vi "Host_XYConstantCurrent.vi"() -> ()   [LabVIEW 2014]
uses:
  <vilib>/FPGAPlugInAG/PCIe-7851R/niLvFpga_Open_PCIe-7851R.vi
  <vilib>/rvi/interface/common/dynamic/niFpgaDynamicAddResources.vi
  <vilib>/Utility/error.llb/Error Cluster From Error Code.vi
  <vilib>/rvi/errors/niLvFpgaAdjustHostInterfaceError.vi
  <vilib>/FPGAPlugInAG/Dynamic/niLvFpga_Close_Dynamic.vi
  <vilib>/rvi/interface/nirviOpenFPGA/nirviOpenFPGA.xnode
  FPGA Bitfiles/PCCrossingXYProj_FPGATarget_FPGAXYMoving_0UyQVClWLPs.lvbitx
  <vilib>/rvi/interface/nirviReadWriteControl/nirviReadWriteControl.xnode
  <vilib>/rvi/interface/nirviCloseFPGA/nirviCloseFPGA.xnode
  NiFpgaLv.dll
  <vilib>/rvi/interface/Simulation/niFpgaSimulationCallBeginRW.vi
panel:
  out "YPresNum":i32
  out "XPresNum":i32
  in  "stop":bool
  in  "YOffset":i16
  in  "XOffset":i16
  in  "YStepLen":i16
  in  "XStepLen":i16
  in  "YNum":i16
  in  "XNum":i16
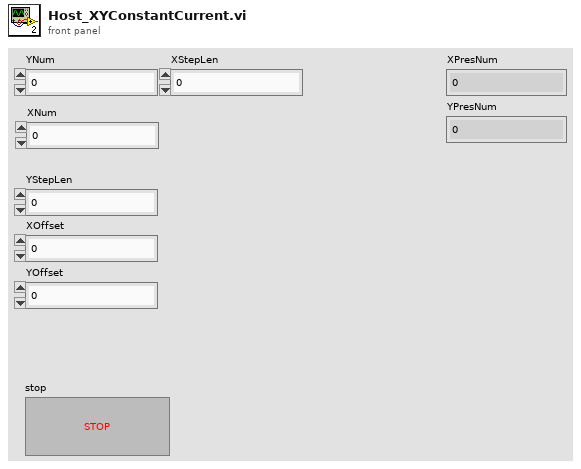
[diagram p1: front panel]
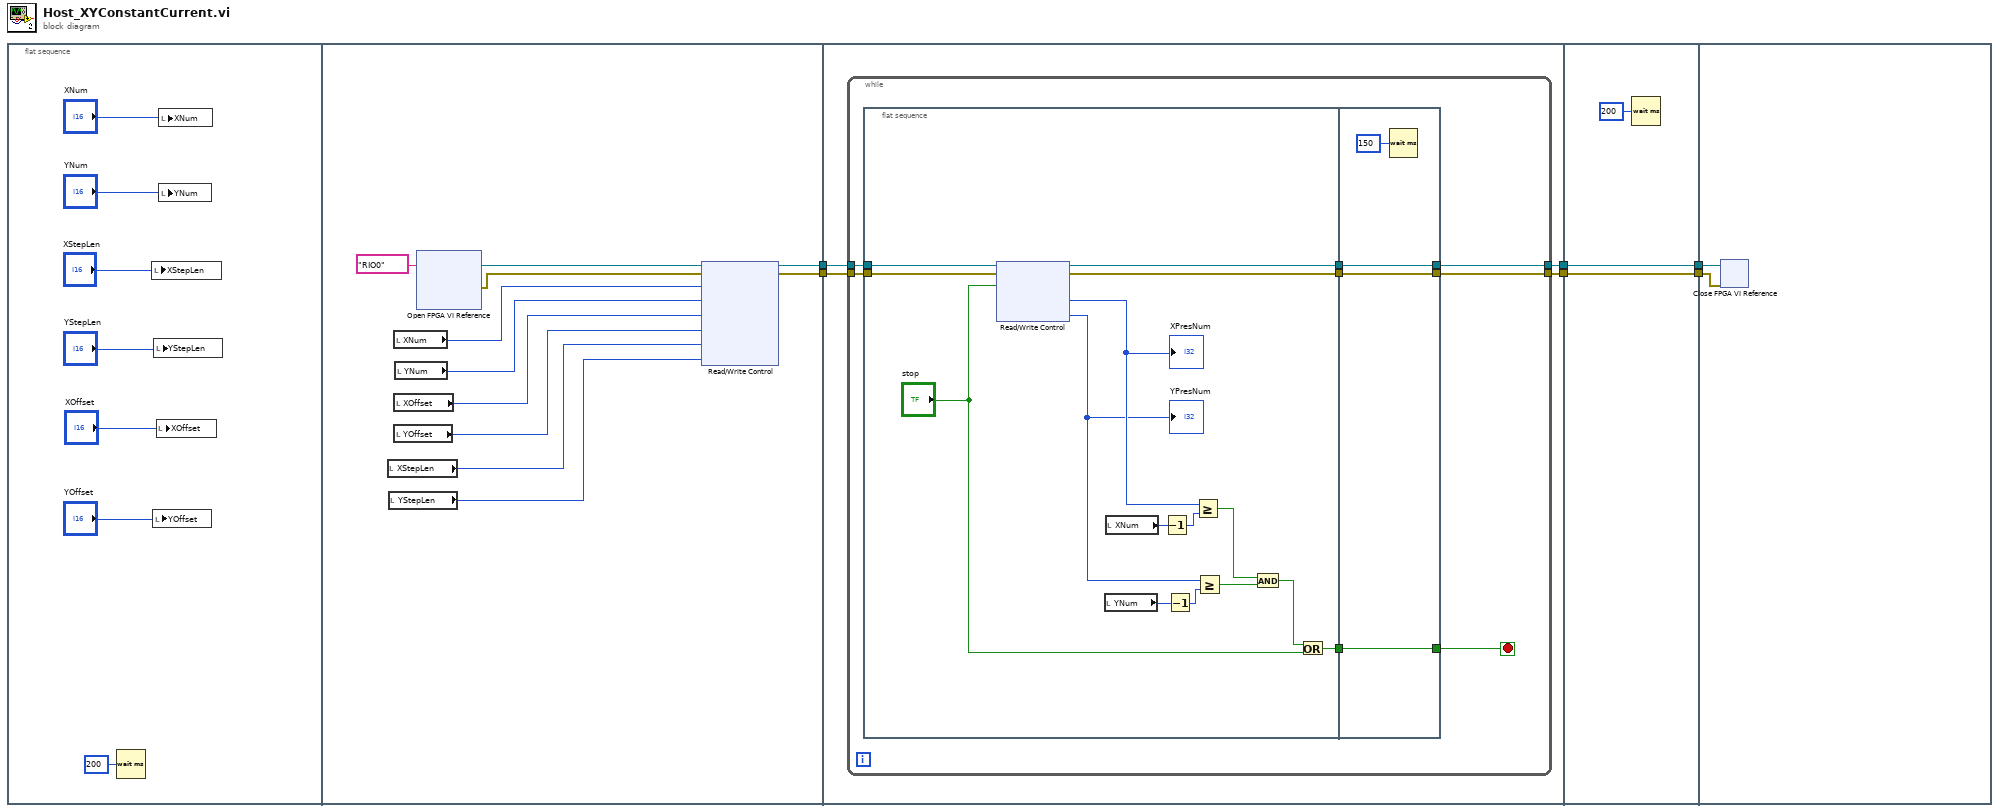
[diagram p0: block diagram]
diagram:
  n1 = flat-sequence {
    tunnel: [w15] -> w6
    tunnel: [w14] -> w5
    tunnel: w6 -> [w28]
    tunnel: w5 -> [w27]
    tunnel: [w26] -> w3
    tunnel: [w25] -> w2
    tunnel: [w57] -> w4
    tunnel: w3 -> [w57]
    tunnel: w2 -> [w56]
    tunnel: [w56] -> w1
    tunnel: w4 -> [w60]
    tunnel: w1 -> [w59]
    frame #0 {
      n2 = Wait (ms)(milliseconds to wait=u32 200) -> ()  [unwired: 1 out]
      n3 = local write "XStepLen"("XStepLen") -> ()
      n4 = local write "YOffset"("YOffset") -> ()
      n5 = local write "YStepLen"("YStepLen") -> ()
      n6 = local write "XOffset"("XOffset") -> ()
      n7 = local write "XNum"("XNum") -> ()
      n8 = local write "YNum"("YNum") -> ()
    }
    frame #1 {
      n9 = local read "XStepLen"() -> (w17:i16)
      n10 = local read "YStepLen"() -> (w16:i16)
      n11 = local read "XNum"() -> (w21:i16)
      n12 = local read "XOffset"() -> (w19:i16)
      n13 = local read "YOffset"() -> (w18:i16)
      n14 = local read "YNum"() -> (w20:i16)
      n15 = xnode "Open FPGA VI Reference"("resource name"=tag "RIO0") -> ("FPGA VI Reference Out"=w23:refnum<k20>, "error out"=w22:errorcluster)  [unwired: 1 in]
      n16 = xnode "Read/Write Control"("FPGA VI Reference In"=w23, "error in"=w22, "XNum"=w21, "YNum"=w20, "XOffset"=w19, "YOffset"=w18, "XStepIndex"=w17, "YStepIndex"=w16) -> ("FPGA VI Reference Out"=w15:refnum<k20>, "error out"=w14:errorcluster)
    }
    frame #2 {
      n17 = while {
        tunnel: w28 -> [w36]
        tunnel: w27 -> [w35]
        tunnel: [w32] -> w26
        tunnel: [w29] -> w25
        stop <- w33 stop-if-true
        n18 = flat-sequence {
          tunnel: w36 -> [w51]
          tunnel: w35 -> [w50]
          tunnel: [w39] -> w34
          tunnel: [w38] -> w31
          tunnel: [w37] -> w30
          tunnel: [w54] -> w33
          tunnel: w34 -> [w54]
          tunnel: [w53] -> w32
          tunnel: w31 -> [w53]
          tunnel: w30 -> [w52]
          tunnel: [w52] -> w29
          frame #0 {
            n19 = xnode "Read/Write Control"("FPGA VI Reference In"=w51, "error in"=w50, "stop"="stop") -> ("FPGA VI Reference Out"=w38:refnum<k20>, "error out"=w37:errorcluster, "XPresNum"=w49:i32, "YPresNum"=w48:i32)
            "XPresNum" <- w49
            "YPresNum" <- w48
            n20 = local read "YNum"() -> (w45:i16)
            n21 = local read "XNum"() -> (w46:i16)
            n22 = Decrement(x=w46) -> (x-1=w47:i16)
            n23 = Decrement(x=w45) -> (x-1=w44:i16)
            n24 = Greater Or Equal?(x=w49, y=w47) -> (x >= y?=w43:bool)
            n25 = Greater Or Equal?(x=w48, y=w44) -> (x >= y?=w42:bool)
            n26 = And(x=w43, y=w42) -> (x .and. y?=w41:bool)
            n27 = Or(x=w41, y="stop") -> (x .or. y?=w39:bool)
          }
          frame #1 {
            n28 = Wait (ms)(milliseconds to wait=u32 150) -> ()  [unwired: 1 out]
          }
        }
      }
    }
    frame #3 {
      n29 = Wait (ms)(milliseconds to wait=u32 200) -> ()  [unwired: 1 out]
    }
    frame #4 {
      n30 = xnode "Close FPGA VI Reference"("FPGA VI Reference In"=w60, "error in"=w59) -> ()  [unwired: 1 out]
    }
  }
